vi "PDC_GetColorTempMode.vi"(0 "DeviceNo":u32, 5 "ChildNo":u32, 11 "error in (no error)":errorcluster) -> (3 "Mode":u32, 4 "ReturnValue":u32, 6 "R":u32, 8 "G":u32, 10 "B":u32, 14 "ErrorCode":u32, 15 "error out":errorcluster)   [LabVIEW 2015]
doc: "This VI retrieves the color temperature status of the specified child device."
uses:
  PDCLIB.dll
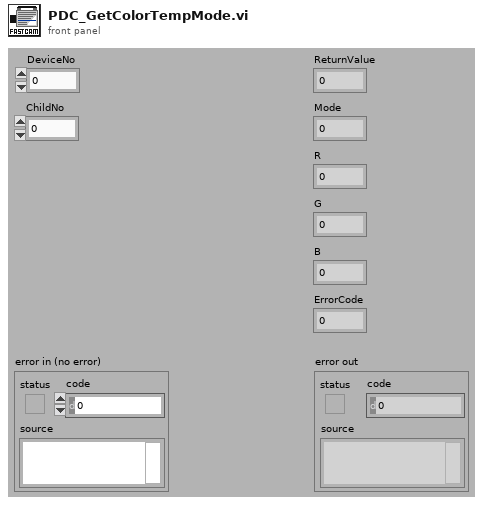
[diagram p1: front panel]
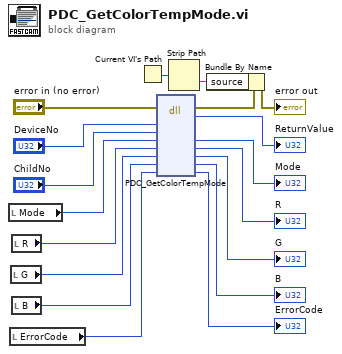
[diagram p0: block diagram]
diagram:
  n1 = local read "Mode"() -> (w12:u32)
  n2 = local read "ErrorCode"() -> (w15:u32)
  n3 = local read "G"() -> (w8:u32)
  n4 = local read "R"() -> (w11:u32)
  n5 = local read "B"() -> (w7:u32)
  n6 = Current VI's Path() -> (path=w3:path)
  n7 = dll-call lib="PDCLIB.dll" fn="PDC_GetColorTempMode"(error in="error in (no error)", "nDeviceNo"="DeviceNo", "nChildNo"="ChildNo", "pMode"=w12, "pR"=w11, "pG"=w8, "pB"=w7, "pErrorCode"=w15) -> (error out=w2:errorcluster, "return type"=→"ReturnValue":u32, "pMode"=→"Mode":u32, "pR"=→"R":u32, "pG"=→"G":u32, "pB"=→"B":u32, "pErrorCode"=→"ErrorCode":u32)  [unwired: 4 in, 1 out]
  n8 = Strip Path(path=w3) -> (name=w4:string)  [unwired: 1 out]
  n9 = Bundle By Name(cluster=w2, "source"=w4) -> (→"error out":errorcluster)
